vi "Create.vi"(6 "Object Name":string, 8 "error in (no error)":errorcluster, 9 "Arguments":string, 10 "Method Name":string, 11 "Response Notifier":refnum<notifier>) -> (0 "error out":errorcluster, 3 "Call out":refnum<class "Call.lvclass">)   [LabVIEW 2013, in "JKI_Python_Bridge_for_LV.lvlib" / "Call.lvclass"]
uses:
  Call.lvclass
  Server/Type Definitions/Python Response - Cluster.ctl
  Call.lvclass/Call.ctl
  Server/Server.lvclass
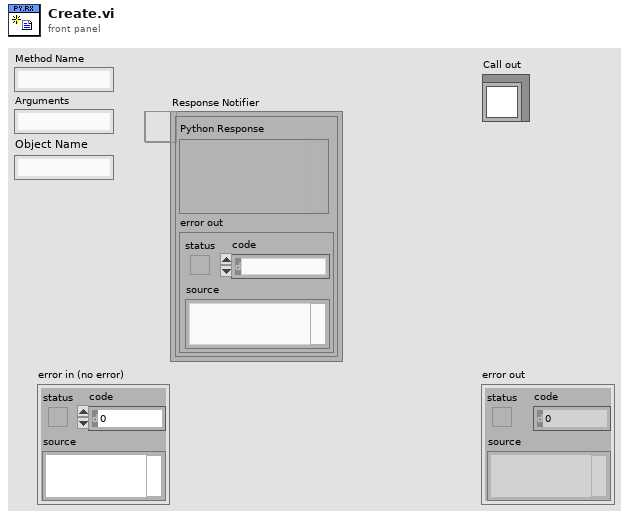
[diagram p1: front panel]
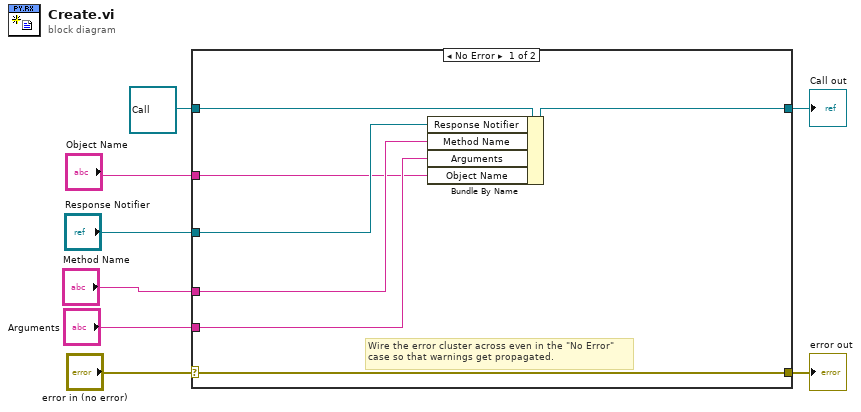
[diagram p0: block diagram]
diagram:
  n1 = case shown="No Error" "error in (no error)" {
    selector: "error in (no error)" -> [w14 w17]
    tunnel: [w14 w17] -> w7
    tunnel: [w13 w16] -> w5
    tunnel: refnum<class "Call.lvclass"> refnum ("Response in") -> [w15 w16]
    tunnel: "Response Notifier" -> [w12 _]
    tunnel: "Method Name" -> [w11 _]
    tunnel: "Arguments" -> [w10 _]
    tunnel: "Object Name" -> [w9 _]
    frame No Error {
      # "Wire the error cluster across even in the \"No Error\"\ncase so that warnings get propagated."
      n2 = Bundle By Name(cluster=w15, "Response Notifier"=w12, "Method Name"=w11, "Arguments"=w10, "Object Name"=w9) -> (w13:refnum<class "Call.lvclass">)
    }
    frame Error {
    }
  }
  "error out" <- w7
  "Call out" <- w5
